vi "FGV_scaling_calibration_points.vi"(7 "Actions":T1(ring), 8 "error in (no error)":errorcluster, 10 "Delete Index":i32, 11 "Data In":sgl[](array[numeric])) -> (0 "error out":errorcluster, 3 "Data Out":dbl[][](array[numeric]))   [LabVIEW 2020]
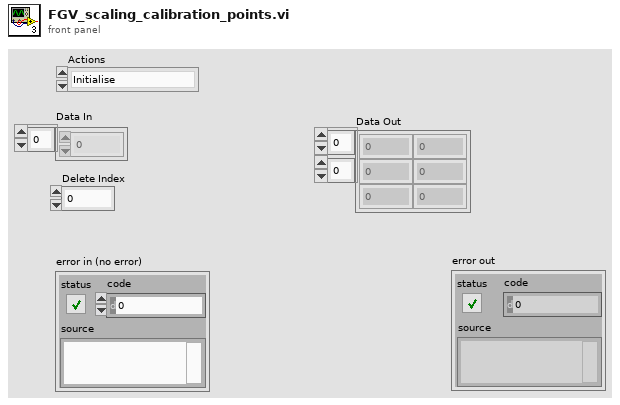
[diagram p1: front panel]
types:
  T1 = enum16{"Initialise", "Add", "Remove", "Read", "Clear"}
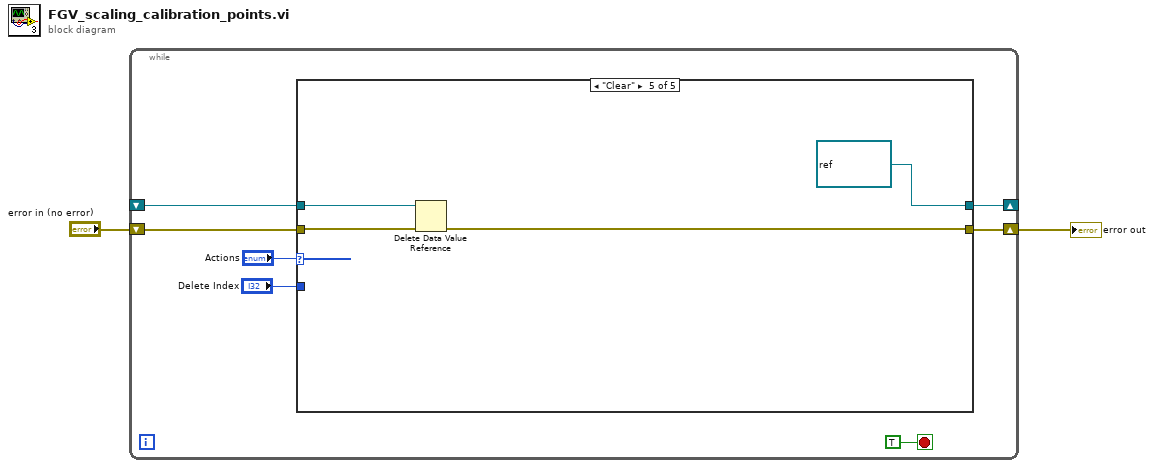
[diagram p0: block diagram]
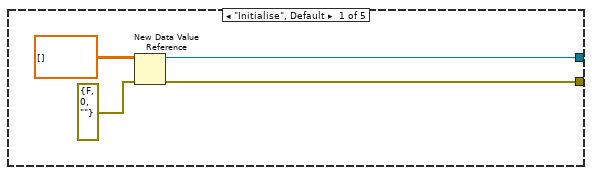
[diagram p2: hidden frame]
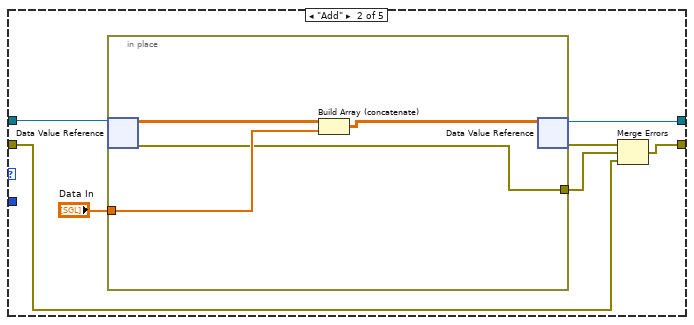
[diagram p3: hidden frame]
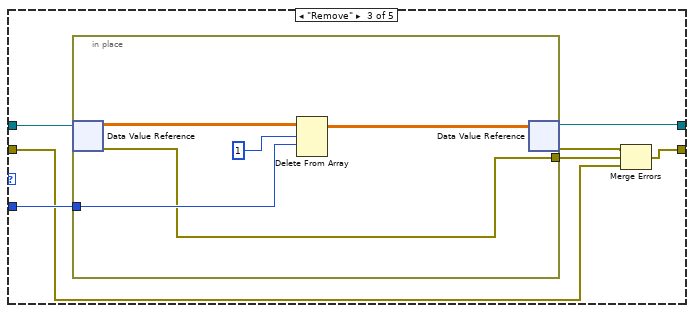
[diagram p4: hidden frame]
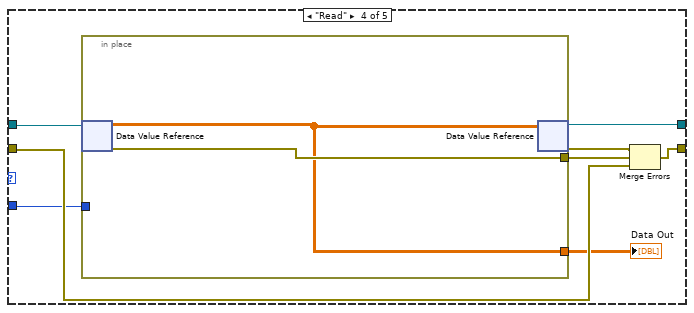
[diagram p5: hidden frame]
diagram:
  n1 = while {
    shift-right: [w8] -> _
    shift-left: _ -> [w7]
    shift-right: [w6] -> w2
    shift-left: "error in (no error)" -> [w5]
    stop <- TRUE stop-if-true
    n2 = case shown="\"Clear\"" "Actions" {
      tunnel: [w12 w19 w29 w39 refnum<data-value> refnum ("data value reference")] -> w8
      tunnel: w7 -> [_ w20 w31 w42 w50]
      tunnel: [w11 w14 w27 w38 w48] -> w6
      tunnel: w5 -> [_ w15 w25 w41 w49]
      tunnel: "Delete Index" -> [_ _ w30 w40 _]
      frame "Initialise", Default {
        n3 = New Data Value Reference(data value=sgl[][] [], error in=errorcluster {"status"=FALSE, "code"=0, "source"=""} ("error in (no error)")) -> (data value reference=w12:refnum<data-value>, error out=w11:errorcluster)
      }
      frame "Add" {
        n4 = in-place {
          in-place-border: "Data In" -> [w22]
          in-place-border: [w21] -> w16
          n5 = in-place-dvr #1(w20) -> (w24:sgl[][], w21:errorcluster)
          n6 = Build Array (concatenate)(w24, w22) -> (w23:sgl[][])
          n7 = in-place-dvr #1(w23) -> (w19:refnum<data-value>, w17:errorcluster)
        }
        n8 = Merge Errors(w17, w16, w15) -> (w14:errorcluster)
      }
      frame "Remove" {
        n9 = in-place {
          in-place-border: w30 -> [w34]
          in-place-border: [w32] -> w26
          n10 = in-place-dvr #2(w31) -> (w36:sgl[][], w32:errorcluster)
          n11 = Delete From Array(array=w36, length=1, index (row)=w34) -> (array with subset deleted=w33:sgl[][])  [unwired: 1 in, 1 out]
          n12 = in-place-dvr #2(w33) -> (w29:refnum<data-value>, w28:errorcluster)
        }
        n13 = Merge Errors(w28, w26, w25) -> (w27:errorcluster)
      }
      frame "Read" {
        n14 = in-place {
          in-place-border: w40 -> [_]
          in-place-border: [w46] -> w43
          in-place-border: [w45] -> w37
          n15 = in-place-dvr #3(w42) -> (w45:sgl[][], w46:errorcluster)
          n16 = in-place-dvr #3(w45) -> (w39:refnum<data-value>, w44:errorcluster)
        }
        "Data Out" <- w37
        n17 = Merge Errors(w44, w43, w41) -> (w38:errorcluster)
      }
      frame "Clear" {
        n18 = Delete Data Value Reference(data value reference=w50, error in=w49) -> (error out=w48:errorcluster)  [unwired: 1 out]
      }
    }
  }
  "error out" <- w2
